vi "Read Button Text.vi"(8 "error in (no error)":errorcluster, 11 "Generic Plugin in":refnum<class "Generic Plugin.lvclass">) -> (0 "error out":errorcluster, 2 "Button Text":string, 3 "Generic Plugin out":refnum<class "Generic Plugin.lvclass">)   [LabVIEW 2011, in "Generic Plugin.lvclass"]
uses:
  Generic Plugin.lvclass
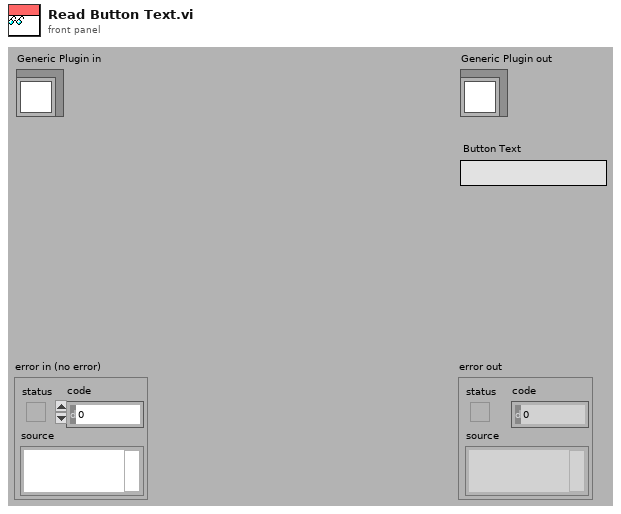
[diagram p1: front panel]
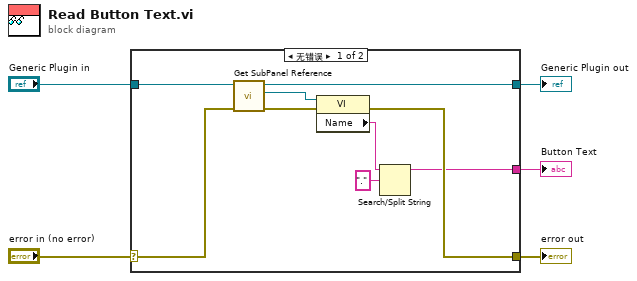
[diagram p0: block diagram]
diagram:
  n1 = case shown="无错误" "error in (no error)" {
    selector: "error in (no error)" -> [w12 w15]
    tunnel: [w10 w15] -> w4
    tunnel: [w9 w16] -> w2
    tunnel: "Generic Plugin in" -> [w11 w16]
    tunnel: [w7 _] -> w1
    frame No Error {
      n2 = call-dynamic "Get SubPanel Reference.vi"("error in (no error)"=w12, "Generic Plugin in"=w11) -> ("error out"=w13:errorcluster, "VI Ref"=w14:refnum<vi>, "Generic Plugin out"=w9:refnum<class "Generic Plugin.lvclass">)  [unwired: 7 in]
      n3 = property class="VI"(reference=w14, error in=w13) -> (error out=w10:errorcluster, "Name"=w8:string)  [unwired: 1 out]
      n4 = Search/Split String(string=w8, search string/char (-)=".") -> (substring before match=w7:string)  [unwired: 1 in, 2 out]
    }
    frame Error {
    }
  }
  "error out" <- w4
  "Generic Plugin out" <- w2
  "Button Text" <- w1
